vi "Init.vi"(8 "error in (no error)":errorcluster, 10 "TSF File Path":path) -> (0 "error out":errorcluster, 3 "TSF Parser out":refnum<class "TSF Parser.lvclass">)   [LabVIEW 2016, in "TSF Parser.lvlib" / "TSF Parser.lvclass"]
uses:
  TSF Parser.lvclass
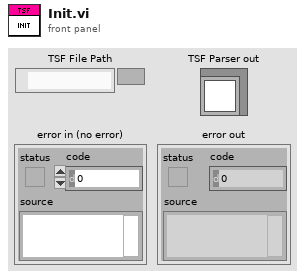
[diagram p1: front panel]
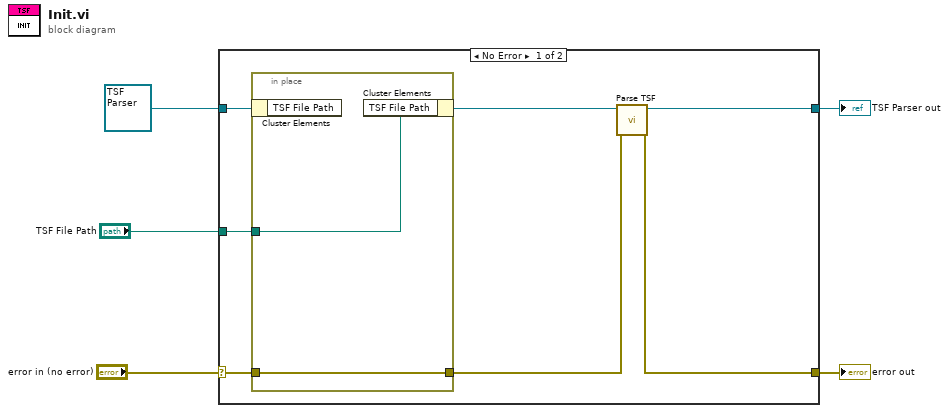
[diagram p0: block diagram]
diagram:
  n1 = case shown="No Error" "error in (no error)" {
    selector: "error in (no error)" -> [w11 w16]
    tunnel: [w8 w16] -> w4
    tunnel: [w6 w15] -> w2
    tunnel: refnum<class "TSF Parser.lvclass"> refnum ("TSF Parser in") -> [w12 w15]
    tunnel: "TSF File Path" -> [w9 _]
    frame No Error {
      n2 = in-place {
        in-place-border: w11 -> [w14]
        in-place-border: [w14] -> w10
        in-place-border: w9 -> [w13]
        n3 = in-place-cluster #1(w12) -> ()  [unwired: 1 out]
        n4 = in-place-cluster #1("TSF File Path"=w13) -> (w7:refnum<class "TSF Parser.lvclass">)
      }
      n5 = call "Parse TSF.vi"("error in (no error)"=w10, "TSF Parser in"=w7) -> ("error out"=w8:errorcluster, "TSF Parser out"=w6:refnum<class "TSF Parser.lvclass">)  [unwired: 8 in]
    }
    frame Error {
    }
  }
  "error out" <- w4
  "TSF Parser out" <- w2
